vi "OSC(Labview v20).vi"() -> ()   [LabVIEW 2021]
uses:
  <vilib>/DAQmx/read.llb/DAQmx Read (Analog DBL 1Chan 1Samp).vi
  <vilib>/DAQmx/create/channels.llb/DAQmx Create Channel (AI-Voltage-Basic).vi
  <vilib>/DAQmx/configure/timing.llb/DAQmx Timing (Sample Clock).vi
  <vilib>/measure/maspectr.llb/FFT Spectrum (Mag-Phase) for 1 Chan.vi
  <vilib>/DAQmx/miscellaneous.llb/DAQmx Fill In Error Info.vi
  <vilib>/measure/NI_MAPro.lvlib
panel:
  in  "Syn_stopREC":bool
  in  "EN_REC":bool
  in  "Syn_Stop":bool
  out "BTN_Stop":bool caption="EN"
  out "fArray":dbl[](array[numeric])
  out "XArray":dbl[](array[numeric])
  out "PageSamples":i32
  in  "Knob 2":i32(knob) scale=0.0..5.0
  in  "采样频率":i32=1000
  in  "Channel":tag
  out "Frequency":cluster{"fArray ":dbl[], "magnitude":dbl[]}(graph)
  in  "EN":bool
  out "Signal":cluster{"XArray":dbl[], dbl[]}(graph)
  # "信号显示系统"
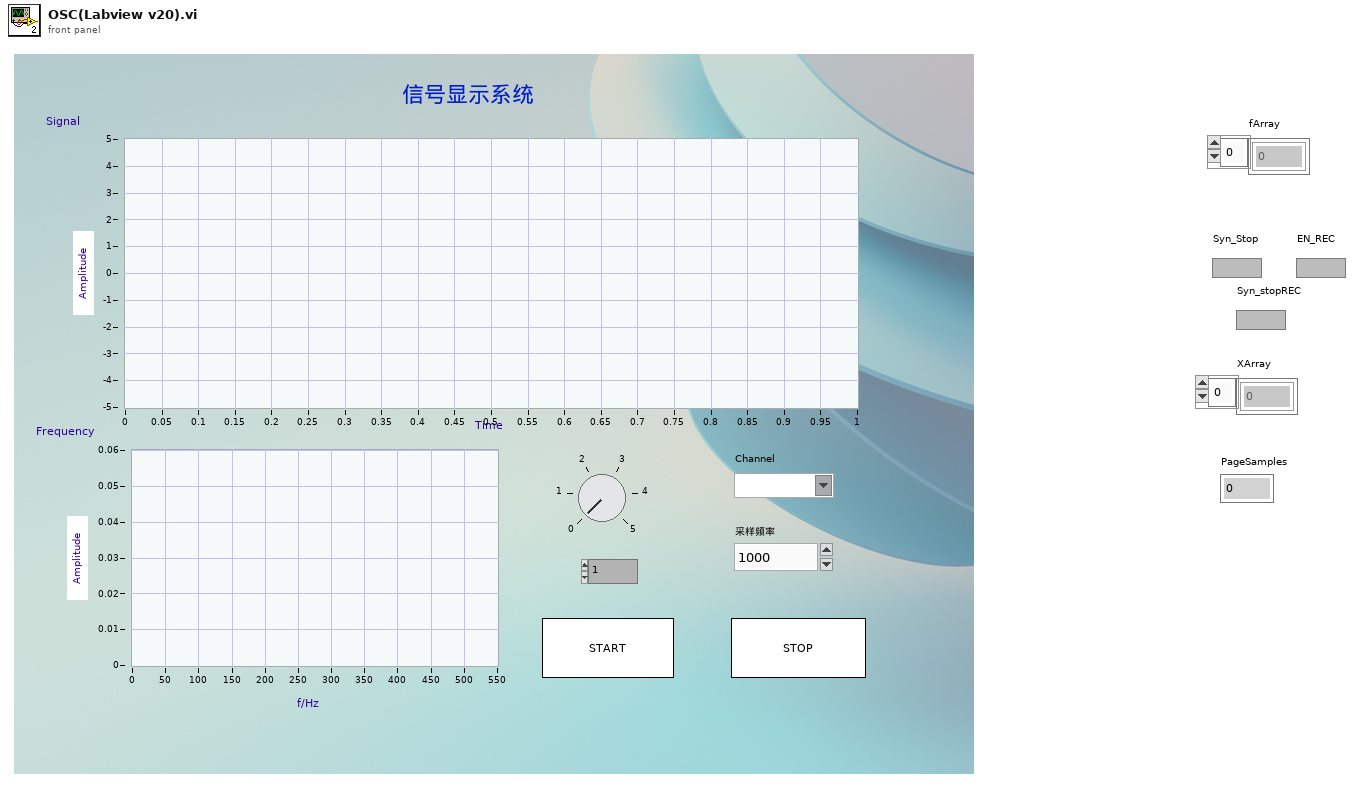
[diagram p1: front panel]
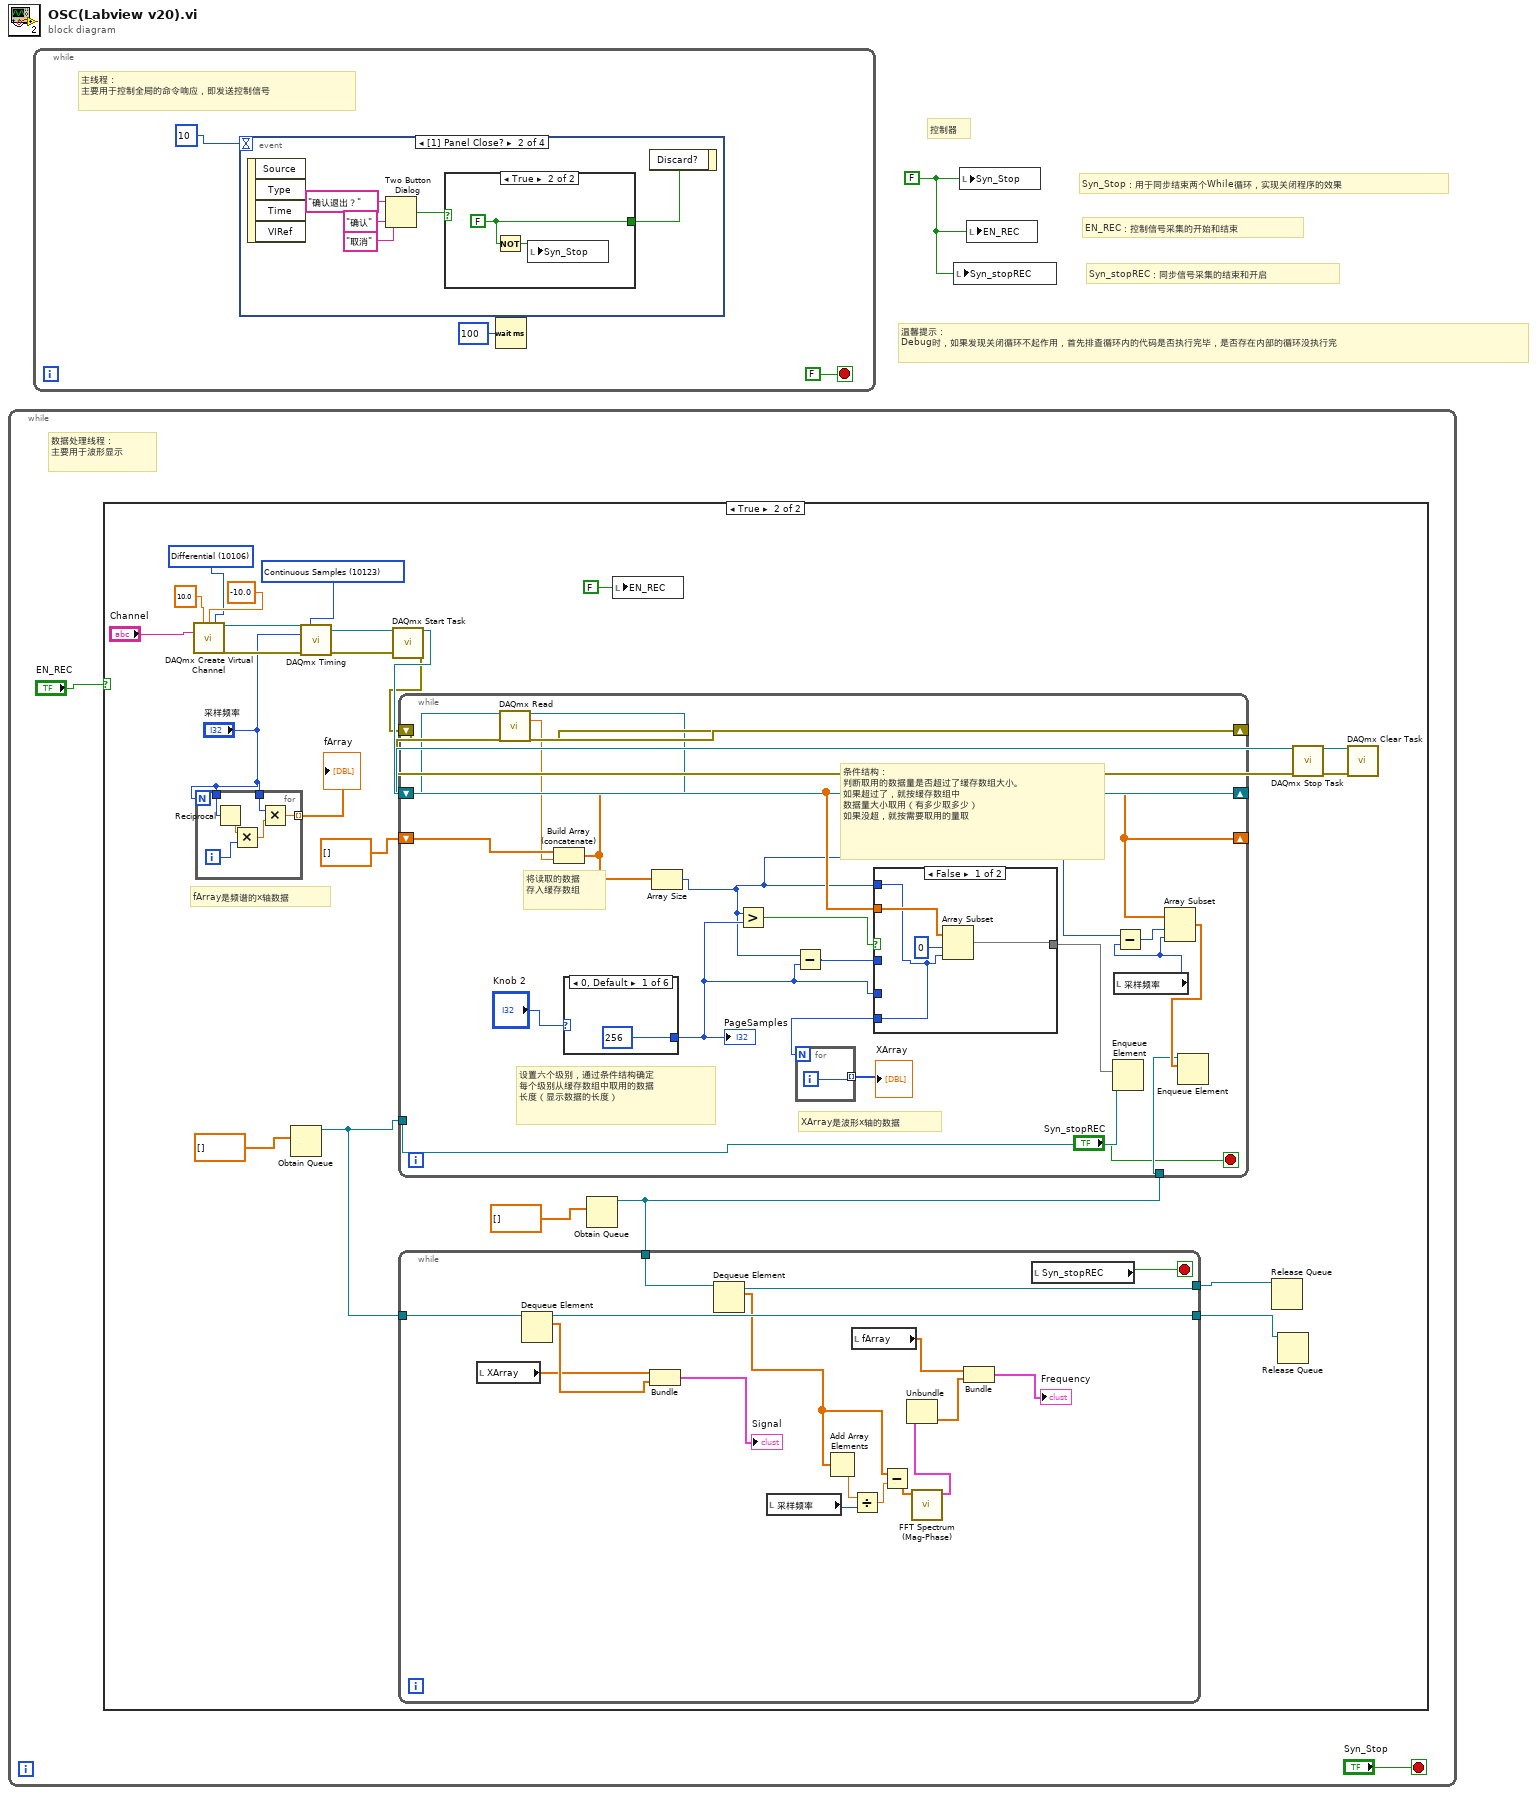
[diagram p0: block diagram]
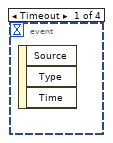
[diagram p2: hidden frame]
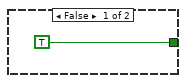
[diagram p3: hidden frame]
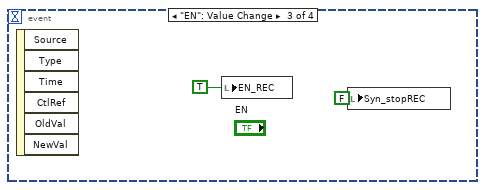
[diagram p4: hidden frame]
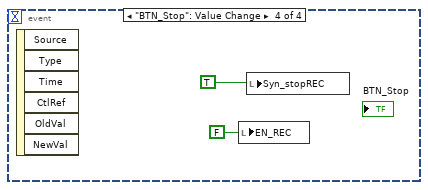
[diagram p5: hidden frame]
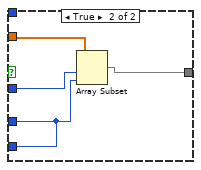
[diagram p7: hidden frame]
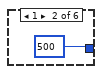
[diagram p8: hidden frame]
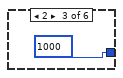
[diagram p9: hidden frame]
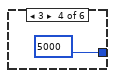
[diagram p10: hidden frame]
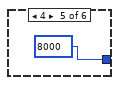
[diagram p11: hidden frame]
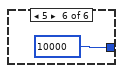
[diagram p12: hidden frame]
diagram:
  w1 = FALSE ("Boolean")
  # "温馨提示：\nDebug时，如果发现关闭循环不起作用，首先排查循环内的代码是否执行完毕，是否存在内部的循环没执行完"
  # "Syn_stopREC：同步信号采集的结束和开启"
  # "EN_REC：控制信号采集的开始和结束"
  # "Syn_Stop：用于同步结束两个While循环，实现关闭程序的效果"
  # "控制器"
  n1 = while {
    stop <- "Syn_Stop" stop-if-true
    # "数据处理线程：\n主要用于波形显示"
    n2 = case shown="True" "EN_REC" {
      frame False {
      }
      frame True {
        w20 = 10123 items=["Finite Samples"=10178, "Continuous Samples"=10123, "Hardware Timed Single Point"=12522] ("sample mode")
        w25 = 10106 items=["Default"=-1, "RSE"=10083, "NRSE"=10078, "Differential"=10106, "Pseudodifferential"=12529] ("input terminal configuration")
        # "fArray是频谱的x轴数据"
        n3 = call-poly <vilib>:"DAQmx Create Virtual Channel.vi"("maximum value"=10.0, "minimum value"=-10.0, "input terminal configuration"=w25, "physical channels"="Channel") -> ("task out"=w24:refnum<k21>, "error out"=w23:errorcluster)  [unwired: 10 in]
        n4 = for {
          N: "采样频率" -> [_]
          tunnel: "采样频率" -> [w34]
          tunnel: "采样频率" -> [w30]
          tunnel: [w29] -> w5 mode=indexing
          i -> [w33]
          n5 = Reciprocal(x=w34) -> (1/x=w32:dbl)
          n6 = Multiply(x=w32, y=w33) -> (x*y=w31:dbl)
          n7 = Multiply(x=w30, y=w31) -> (x*y=w29:dbl)
        }
        "fArray" <- w5
        n8 = Obtain Queue(element data type=dbl[] []) -> (queue out=w10:refnum<queue>)  [unwired: 4 in, 2 out]
        n9 = call-poly <vilib>:"DAQmx Timing.vi"("task/channels in"=w24, "sample mode"=w20, "rate"="采样频率", "error in"=w23) -> ("task out"=w21:refnum<k21>, "error out"=w22:errorcluster)  [unwired: 10 in]
        n10 = call <vilib>:"DAQmx Start Task.vi"("task/channels in"=w21, "error in"=w22) -> ("task out"=w19:refnum<k21>, "error out"=w18:errorcluster)  [unwired: 12 in]
        n11 = Obtain Queue(element data type=dbl[] []) -> (queue out=w8:refnum<queue>)  [unwired: 4 in, 2 out]
        n12 = while {
          shift-right: [w67] -> w14
          shift-left: w19 -> [w72]
          shift-right: [w68] -> w13
          shift-left: w18 -> [w71]
          shift-right: [w58] -> _
          shift-left: dbl[] [] -> [w70]
          tunnel: w10 -> [w65]
          tunnel: w8 -> [w53]
          stop <- "Syn_stopREC" stop-if-true
          # "条件结构：\n判断取用的数据量是否超过了缓存数组大小。\n如果超过了，就按缓存数组中\n数据量大小取用（有多少取多少）\n如果没超，就按需要取用的量取"
          # "XArray是波形x轴的数据"
          # "设置六个级别，通过条件结构确定\n每个级别从缓存数组中取用的数据\n长度（显示数据的长度）"
          # "将读取的数据\n存入缓存数组"
          n13 = call-poly <vilib>:"DAQmx Read.vi"("task/channels in"=w72, "error in"=w71) -> ("task out"=w67:refnum<k21>, "data"=w69:dbl, "error out"=w68:errorcluster)  [unwired: 11 in]
          n14 = Build Array (concatenate)(w70, w69) -> (w58:dbl[])
          n15 = case shown="0, Default" "Knob 2" {
            tunnel: [256 500 1000 5000 8000 10000] -> w61
            frame 0, Default {
            }
            frame 1 {
            }
            frame 2 {
            }
            frame 3 {
            }
            frame 4 {
            }
            frame 5 {
            }
          }
          "PageSamples" <- w61
          n16 = Array Size(array=w58) -> (size(s)=w57:i32)
          n17 = Greater?(x=w57, y=w61) -> (0:w63:bool)
          n18 = Subtract(x=w57, y=w61) -> (x-y=w62:i32)
          n19 = case shown="False" w63 {
            tunnel: [w74 w80] -> w60
            tunnel: w58 -> [w75 w79]
            tunnel: w62 -> [_ w78]
            tunnel: w61 -> [_ w77]
            tunnel: w57 -> [w73 _]
            tunnel: [w73 w77] -> w59
            frame False {
              n20 = Array Subset(array=w75, index=0, length=w73) -> (w74:dbl[])
            }
            frame True {
              n21 = Array Subset(array=w79, index=w78, length=w77) -> (w80:dbl[])
            }
          }
          n22 = for {
            N: w59 -> [_]
            tunnel: [w81] -> w64 mode=indexing
            i -> [w81]
          }
          "XArray" <- w64
          n23 = Enqueue Element(queue=w65, element=w60) -> ()  [unwired: 2 in, 3 out]
          n24 = local read "采样频率"() -> (w55:i32)
          n25 = Subtract(x=w57, y=w55) -> (x-y=w56:i32)
          n26 = Array Subset(array=w58, index=w56, length=w55) -> (w54:dbl[])
          n27 = Enqueue Element(queue=w53, element=w54) -> ()  [unwired: 2 in, 3 out]
        }
        n28 = while {
          tunnel: [w51] -> w11
          tunnel: w10 -> [w50]
          tunnel: w8 -> [w49]
          tunnel: [w48] -> w7
          stop <- w38 stop-if-true
          n29 = local read "XArray"() -> (w36:dbl[])
          n30 = Dequeue Element(queue=w50) -> (queue out=w51:refnum<queue>, element=w37:dbl[])  [unwired: 2 in, 2 out]
          n31 = Bundle("XArray"=w36, w37) -> (→"Signal":cluster{"XArray":dbl[], dbl[]})  [unwired: 1 in]
          n32 = Dequeue Element(queue=w49) -> (queue out=w48:refnum<queue>, element=w44:dbl[])  [unwired: 2 in, 2 out]
          n33 = local read "采样频率"() -> (w40:i32)
          n34 = Add Array Elements(numeric array=w44) -> (sum=w43:dbl)
          n35 = local read "fArray"() -> (w39:dbl[])
          n36 = Divide(x=w43, y=w40) -> (x/y=w42:dbl)
          n37 = Subtract(x=w44, y=w42) -> (x-y=w41:dbl[])
          n38 = call-poly <vilib>:"FFT Spectrum (Mag-Phase).vi"("time signal"=w41) -> ("magnitude"=w47:cluster{"f0":dbl, "df":dbl, "magnitude":dbl[]})  [unwired: 6 in, 4 out]
          n39 = Unbundle(w47) -> ("magnitude"=w45:dbl[])  [unwired: 2 out]
          n40 = Bundle("fArray"=w39, "magnitude"=w45) -> (→"Frequency":cluster{"fArray ":dbl[], "magnitude":dbl[]})  [unwired: 1 in]
          n41 = local read "Syn_stopREC"() -> (w38:bool)
        }
        n42 = local write "EN_REC"(FALSE ("Boolean 2")) -> ()
        n43 = Release Queue(queue=w7) -> ()  [unwired: 2 in, 3 out]
        n44 = Release Queue(queue=w11) -> ()  [unwired: 2 in, 3 out]
        n45 = call <vilib>:"DAQmx Stop Task.vi"("task/channels in"=w14, "error in"=w13) -> ("task out"=w17:refnum<k21>, "error out"=w16:errorcluster)  [unwired: 12 in]
        n46 = call <vilib>:"DAQmx Clear Task.vi"("task in"=w17, "error in"=w16) -> ()  [unwired: 13 in, 1 out]
      }
    }
  }
  n47 = while {
    stop <- FALSE stop-if-true
    # "主线程：\n主要用于控制全局的命令响应，即发送控制信号"
    n48 = event shown="[1] Panel Close?" {
      selector: _ -> [_ _ _ _]
      dyn-events: _ -> [_ _ _ _]
      timeout: 10 -> [_ _ _ _]
      event Timeout {
        n49 = event-data() -> ()  [unwired: 1 in, 3 out]
      }
      event Panel Close? {
        n50 = event-data() -> ()  [unwired: 1 in, 4 out]
        n51 = Two Button Dialog(message="确认退出？", 1:"取消" ("F button name (\"Cancel\")"), 2:"确认" ("T button name (\"OK\")")) -> (T button?=w92:bool)
        n52 = case shown="True" w92 {
          tunnel: [TRUE w98] -> w91
          frame False {
          }
          frame True {
            w98 = FALSE
            n53 = Not(x=w98) -> (.not. x?=w97:bool)
            n54 = local write "Syn_Stop"(w97) -> ()
          }
        }
        n55 = event-data("Discard?"=w91) -> ()  [unwired: 1 in, 1 out]
      }
      event "EN": Value Change {
        n56 = event-data() -> ()  [unwired: 1 in, 6 out]
        n57 = local write "EN_REC"(TRUE ("Boolean 2")) -> ()
        n58 = local write "Syn_stopREC"(FALSE ("Boolean 3")) -> ()
      }
      event "BTN_Stop": Value Change {
        n59 = event-data() -> ()  [unwired: 1 in, 6 out]
        n60 = local write "EN_REC"(FALSE ("Boolean 2")) -> ()
        n61 = local write "Syn_stopREC"(TRUE ("Boolean 3")) -> ()
      }
    }
    n62 = Wait (ms)(milliseconds to wait=u32 100) -> ()  [unwired: 1 out]
  }
  n63 = local write "Syn_stopREC"(w1) -> ()
  n64 = local write "Syn_Stop"(w1) -> ()
  n65 = local write "EN_REC"(w1) -> ()
